vi "Compute Distance.vi"(8 "Y Image Resolution":i32, 9 "X Image Resolution":i32, 10 "Bounding Box":T1, 11 "Camera Type":enum16{"206", "1011"}(ring)) -> (2 "Target Center (-1 to 1)":cluster{"X":dbl, "Y":dbl}, 3 "Distance (ft)":dbl)   [LabVIEW 2012]
doc: "Using the camera lens information and the real world width of the target, determine the distance to the target."
panel:
  in  "Camera view angle":dbl[](array[numeric])=[48.0, 43.5]
  # "Axis 206\nAxis M1011"
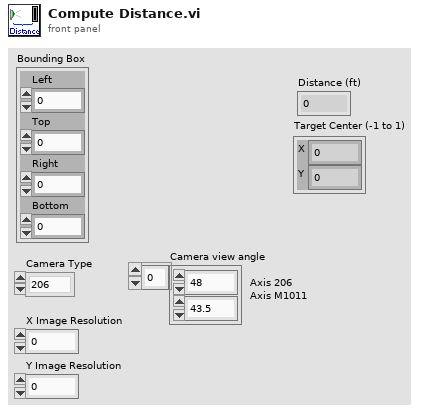
[diagram p1: front panel]
types:
  T1 = cluster{"Left":dbl, "Top":dbl, "Right":dbl, "Bottom":dbl}
  T2 = cluster{"X Image Resolution":i32, "Y Image Resolution":i32}
  T3 = cluster{"X Image Resolution":dbl, "Y Image Resolution":dbl}
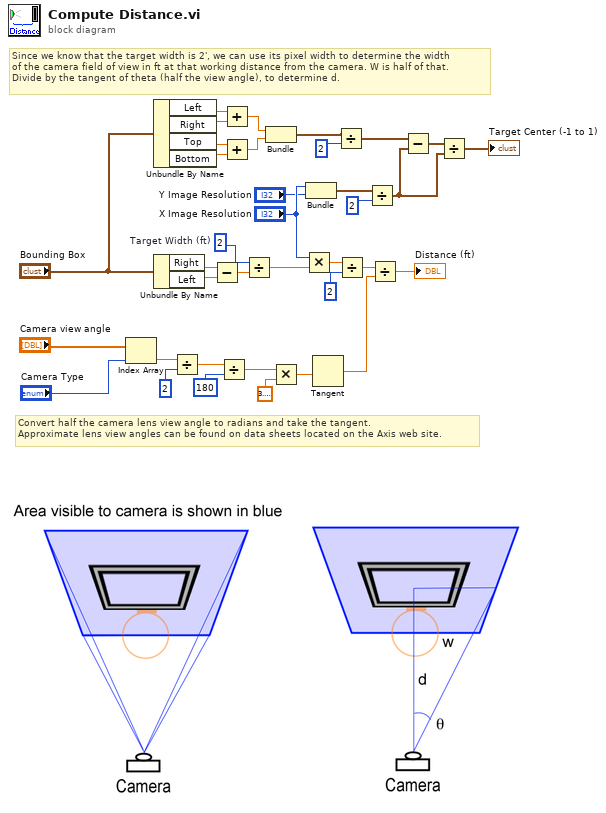
[diagram p0: block diagram]
diagram:
  w18 = 2  # Target Width (ft)
  # "Convert half the camera lens view angle to radians and take the tangent.\nApproximate lens view angles can be found on data sheets located on the Axis web site."
  # "Since we know that the target width is 2', we can use its pixel width to determine the width\nof the camera field of view in ft at that working distance from the camera. W is half of that.\nDivide by the tangent of theta (half the view angle), to determine d."
  n1 = Index Array(array="Camera view angle", index="Camera Type") -> (element=w32:dbl)
  n2 = Unbundle By Name("Bounding Box") -> ("Left"=w13:dbl, "Right"=w14:dbl, "Top"=w16:dbl, "Bottom"=w15:dbl)
  n3 = Unbundle By Name("Bounding Box") -> ("Right"=w22:dbl, "Left"=w21:dbl)
  n4 = Divide(x=w32, y=2) -> (x/y=w29:dbl)
  n5 = Subtract(x=w22, y=w21) -> (x-y=w20:dbl)
  n6 = Divide(x=w29, y=180) -> (x/y=w28:dbl)
  n7 = Add(x=w13, y=w14) -> (x+y=w11:dbl)
  n8 = Add(x=w16, y=w15) -> (x+y=w10:dbl)
  n9 = Divide(x=w18, y=w20) -> (x/y=w19:dbl)
  n10 = Bundle(w11, w10) -> (w5:cluster{dbl, dbl})  [unwired: 1 in]
  n11 = Multiply(x=w28, y=3.141592653589793) -> (x*y=w30:dbl)
  n12 = Multiply(x="X Image Resolution", y=w19) -> (x*y=w23:dbl)
  n13 = Bundle("X Image Resolution"="X Image Resolution", "Y Image Resolution"="Y Image Resolution") -> (w7:T2)  [unwired: 1 in]
  n14 = Tangent(1:w30) -> (0:w36:dbl)
  n15 = Divide(x=w5, y=2) -> (x/y=w4:cluster{dbl, dbl})
  n16 = Divide(x=w23, y=2) -> (x/y=w25:dbl)
  n17 = Divide(x=w7, y=2) -> (x/y=w2:T3)
  n18 = Divide(x=w25, y=w36) -> (x/y=→"Distance (ft)":dbl)
  n19 = Subtract(x=w4, y=w2) -> (x-y=w3:cluster{dbl, dbl})
  n20 = Divide(x=w3, y=w2) -> (x/y=→"Target Center (-1 to 1)":cluster{dbl, dbl})
